vi "Msg Loop.vi"(11 "LVCAM in":refnum<class "LVCAM.lvclass">) -> ()   [LabVIEW 2021, in "LVCAM.lvlib" / "LVCAM.lvclass"]
uses:
  LVCAM.lvclass
  Msg/Msg.lvclass
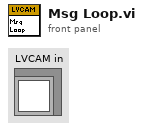
[diagram p1: front panel]
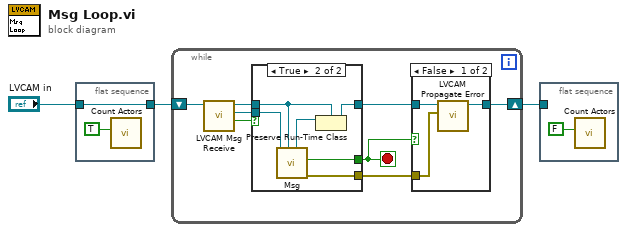
[diagram p0: block diagram]
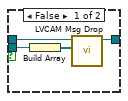
[diagram p3: hidden frame]
diagram:
  n1 = flat-sequence {
    tunnel: [w4] -> w2
    tunnel: "LVCAM in" -> [w4]
    frame #0 {
      n2 = call "Count Actors.vi"("Increment?"=TRUE) -> ()  [unwired: 11 in]
    }
  }
  n3 = while {
    shift-right: [w13] -> w1
    shift-left: w2 -> [w7]
    stop <- w8 stop-if-true
    n4 = call-dynamic "LVCAM Msg Receive.vi"("LVCAM Msg Receive in"=w7) -> ("DeQ Msg?"=w10:bool, "Msg"=w11:refnum<class "Msg.lvclass">, "LVCAM Msg Receive out"=w6:refnum<class "LVCAM.lvclass">)  [unwired: 8 in]
    n5 = case shown="True" w10 {
      tunnel: w6 -> [w21 w27]
      tunnel: [_ w26] -> w9
      tunnel: [_ w22] -> w8
      tunnel: [w18 w25] -> w12
      tunnel: w11 -> [w20 w23]
      frame False {
        n6 = Build Array(w20) -> (w19:refnum<class "Msg.lvclass">[])
        n7 = call-dynamic "LVCAM Msg Drop.vi"("Remaining Elements"=w19, "LVCAM Msg Drop in"=w21) -> ("LVCAM Msg Drop out"=w18:refnum<class "LVCAM.lvclass">)  [unwired: 9 in]
      }
      frame True {
        n8 = call-dynamic "Msg.vi"("LVCAM in"=w27, "Msg in"=w23) -> ("error out"=w26:errorcluster, "Destroyed Self?"=w22:bool, "LVCAM out"=w24:refnum<class "LVCAM.lvclass">)  [unwired: 7 in]
        n9 = Preserve Run-Time Class(object in=w24, 2:w27) -> (object out=w25:refnum<class "LVCAM.lvclass">)  [unwired: 1 in, 1 out]
      }
    }
    n10 = case shown="False" w8 {
      tunnel: [w16 w17] -> w13
      tunnel: w12 -> [w15 w17]
      tunnel: w9 -> [w14 _]
      frame False {
        n11 = call-dynamic "LVCAM Propagate Error.vi"("Error"=w14, "LVCAM Propagate Error in"=w15) -> ("LVCAM Propagate Error out"=w16:refnum<class "LVCAM.lvclass">)  [unwired: 9 in]
      }
      frame True {
      }
    }
  }
  n12 = flat-sequence {
    tunnel: w1 -> [_]
    frame #0 {
      n13 = call "Count Actors.vi"("Increment?"=FALSE) -> ()  [unwired: 11 in]
    }
  }
